vi "Read Charge Pump.vi"(8 "error in (no error)":errorcluster, 11 "Toggle 7.1 in":refnum<class "Toggle 7.1.lvclass">) -> (0 "error out":errorcluster, 2 "Parameter Cluster":T1, 3 "Toggle 7.1 out":refnum<class "Toggle 7.1.lvclass">)   [LabVIEW 2020, in "Toggle 7.1.lvclass"]
uses:
  Toggle 7.1.lvclass
  Controls/Parameter Cluster.ctl
  Toggle 7.1.lvclass/Toggle 7.1.ctl
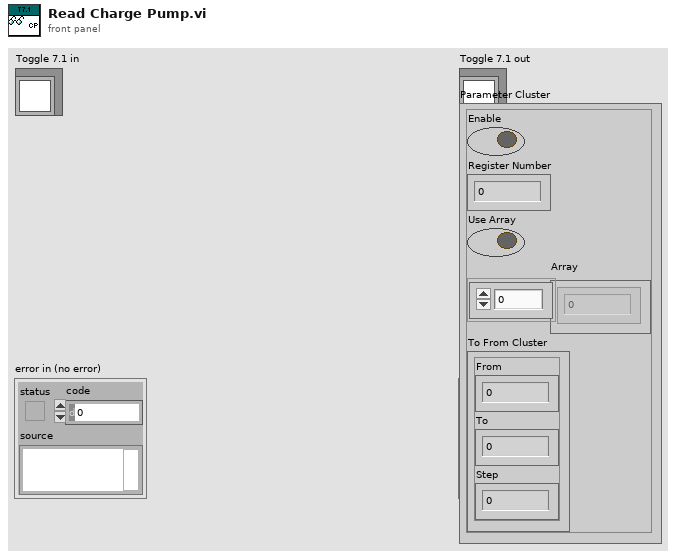
[diagram p1: front panel]
types:
  T1 = typedef "Toggle 7.1.lvclass/Parameter Cluster.ctl" = cluster{"Enable":bool, "Register Number":u32, "Use Array":bool, "Array":dbl[], "To From Cluster":cluster{"From":dbl, "To":dbl, "Step":dbl}}
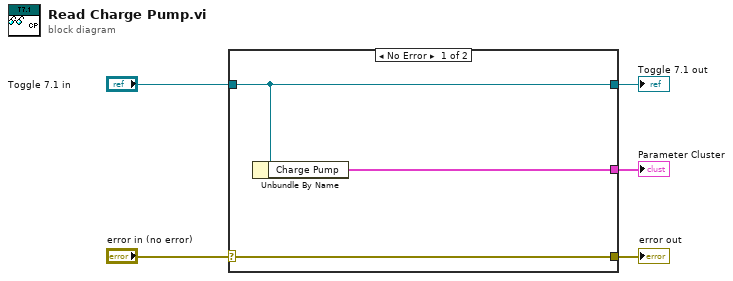
[diagram p0: block diagram]
diagram:
  n1 = case shown="No Error" "error in (no error)" {
    selector: "error in (no error)" -> [w8 w9]
    tunnel: [w8 w9] -> w4
    tunnel: [w7 w10] -> w2
    tunnel: "Toggle 7.1 in" -> [w7 w10]
    tunnel: [w6 _] -> w1
    frame No Error {
      n2 = Unbundle By Name(w7) -> ("Charge Pump"=w6:T1)
    }
    frame Error {
    }
  }
  "error out" <- w4
  "Toggle 7.1 out" <- w2
  "Parameter Cluster" <- w1
